vi "Set Size.vi"(10 "size":u64 format="%d bytes", 11 "Pointer in":refnum<class "Pointer.lvclass">) -> (3 "Pointer out":refnum<class "Pointer.lvclass">)   [LabVIEW 2020, in "Memory Manager.lvlib" / "Pointer.lvclass"]
uses:
  Pointer.lvclass
  Pointer.lvclass/Pointer.ctl
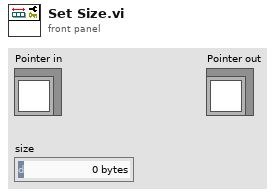
[diagram p1: front panel]
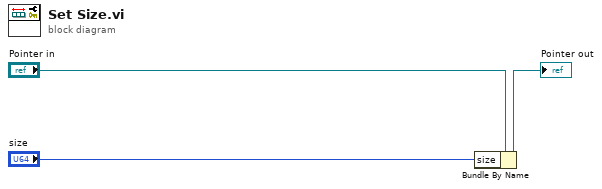
[diagram p0: block diagram]
diagram:
  n1 = Bundle By Name(cluster="Pointer in", "size"="size") -> (→"Pointer out":refnum<class "Pointer.lvclass">)
